vi "Salience Function.vi"(7 "Frequency Axis Scale Factor":dbl, 9 "Time Axis Scale Factor":dbl, 10 "Output STFT":dbl[][](array[numeric])) -> (0 "Time axis":dbl[](array[numeric]), 1 "Peaks Frequencies":dbl[](array[numeric]), 2 "Salience Peaks":dbl[](array[numeric]), 4 "Peak Magnitudes":dbl[](array[numeric]))   [LabVIEW 2014, in "Melody Extraction.lvlib"]
uses:
  Melody Extraction.lvlib
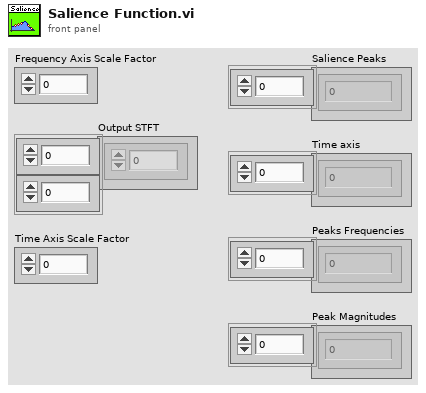
[diagram p1: front panel]
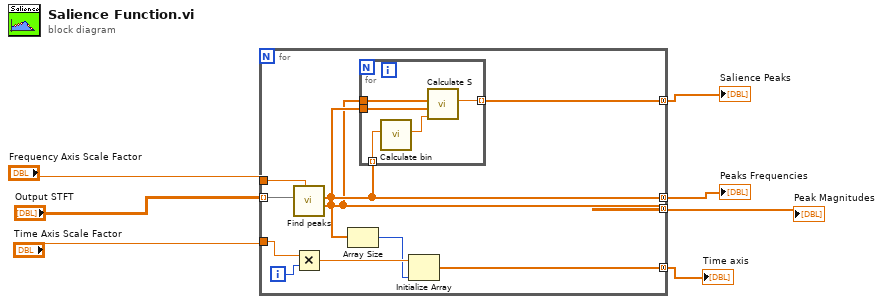
[diagram p0: block diagram]
diagram:
  n1 = for {
    tunnel: "Output STFT" -> [w17] mode=indexing
    tunnel: "Frequency Axis Scale Factor" -> [w16]
    tunnel: "Time Axis Scale Factor" -> [w15]
    tunnel: [w10] -> w5 mode=concatenating
    tunnel: [w8] -> w3 mode=concatenating
    tunnel: [w11] -> w4 mode=concatenating
    tunnel: [w9] -> w6 mode=concatenating
    i -> [w14]
    n2 = call "Find peaks.vi"("Frequency Axis Scale Factor"=w16, "FFT (single frame)"=w17) -> ("Peak Magnitudes"=w8:dbl[], "Peaks Frequencies"=w10:dbl[])  [unwired: 8 in]
    n3 = Multiply(x=w15, y=w14) -> (x*y=w13:dbl)
    n4 = Array Size(array=w8) -> (size(s)=w12:i32)
    n5 = for {
      tunnel: w8 -> [w21]
      tunnel: w10 -> [w20]
      tunnel: w10 -> [w19] mode=indexing
      tunnel: [w18] -> w9 mode=indexing
      n6 = call "Calculate bin.vi"("Frequency"=w19) -> ("B"=w22:dbl)  [unwired: 10 in]
      n7 = call "Calculate S.vi"("Frequency Bin (b)"=w22, "Peak Frequencies"=w20, "Peak Amplitudes"=w21) -> ("S"=w18:dbl)  [unwired: 8 in]
    }
    n8 = Initialize Array(w13, w12) -> (w11:dbl[])
  }
  "Salience Peaks" <- w6
  "Peaks Frequencies" <- w5
  "Time axis" <- w4
  "Peak Magnitudes" <- w3
